vi "readInAoXML.vi"(8 "error in (no error)":errorcluster, 10 "NativeXML in":refnum<class "NativeXML.lvclass">, 11 "deviceDataBase in":refnum<class "deviceDataBase.lvclass">) -> (0 "error out":errorcluster, 1 "device.lvclass out":refnum<class "device.lvclass">, 3 "deviceDataBase out":refnum<class "deviceDataBase.lvclass">)   [LabVIEW 2011, in "Tools.lvlib" / "DatabaseHelpers.lvlib" / "deviceDataBase.lvclass"]
uses:
  deviceDataBase.lvclass
  NativeXML/NativeXML.lvclass
  Database Objects/device/device.lvclass
  Database Objects/device/AnalogDevice/AnalogDevice.lvclass
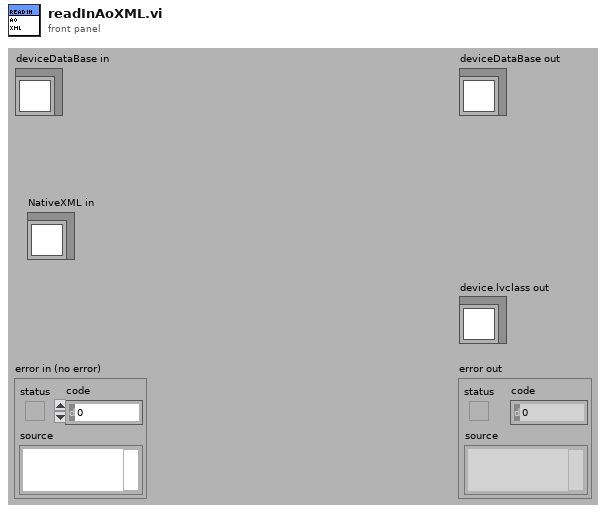
[diagram p1: front panel]
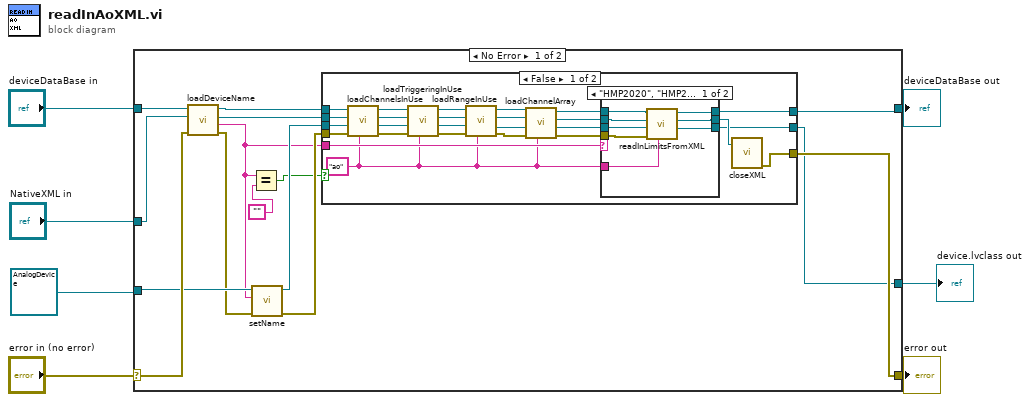
[diagram p0: block diagram]
diagram:
  n1 = case shown="No Error" "error in (no error)" {
    selector: "error in (no error)" -> [w21 w64]
    tunnel: [w13 w64] -> w6
    tunnel: [w12 w63] -> w4
    tunnel: "deviceDataBase in" -> [w22 w63]
    tunnel: "NativeXML in" -> [w20 _]
    tunnel: refnum<class "AnalogDevice.lvclass"> refnum ("Tools.lvlib:DatabaseHelpers.lvlib:AnalogDevice.lvclass") -> [w19 _]
    tunnel: [w9 _] -> w1
    frame No Error {
      n2 = call "loadDeviceName.vi"("error in (no error)"=w21, "NativeXML in"=w20, "deviceDataBase in"=w22) -> ("error out"=w18:errorcluster, "deviceName"=w8:string, "NativeXML out"=w15:refnum<class "NativeXML.lvclass">, "deviceDataBase out"=w17:refnum<class "deviceDataBase.lvclass">)  [unwired: 5 in]
      n3 = Equal?(x=w8, y="") -> (x = y?=w11:bool)
      n4 = call "setName.vi"("error in (no error)"=w18, "name"=w8, "device.lvclass in"=w19) -> ("error out"=w16:errorcluster, "device.lvclass out"=w14:refnum<class "AnalogDevice.lvclass">)  [unwired: 7 in]
      n5 = case shown="False" w11 {
        tunnel: w17 -> [w48 w62]
        tunnel: w16 -> [w47 w60]
        tunnel: w15 -> [w46 _]
        tunnel: w14 -> [w45 w61]
        tunnel: [w32 w60] -> w13
        tunnel: [w26 w61] -> w9
        tunnel: [w31 w62] -> w12
        tunnel: w8 -> [w25 _]
        frame False {
          w23 = "ao"
          n6 = call "loadChannelsInUse.vi"("type"=w23, "error in (no error)"=w47, "device.lvclass"=w45, "NativeXML in"=w46, "deviceDataBase in"=w48) -> ("error out"=w44:errorcluster, "device.lvclass out"=w41:refnum<class "device.lvclass">, "NativeXML out"=w42:refnum<class "NativeXML.lvclass">, "deviceDataBase out"=w43:refnum<class "deviceDataBase.lvclass">)  [unwired: 3 in]
          n7 = call "loadTriggeringInUse.vi"("type"=w23, "error in (no error)"=w44, "device.lvclass"=w41, "NativeXML in"=w42, "deviceDataBase in"=w43) -> ("error out"=w37:errorcluster, "device.lvclass out"=w38:refnum<class "device.lvclass">, "NativeXML out"=w39:refnum<class "NativeXML.lvclass">, "deviceDataBase out"=w40:refnum<class "deviceDataBase.lvclass">)  [unwired: 3 in]
          n8 = call "loadRangeInUse.vi"("type"=w23, "error in (no error)"=w37, "device.lvclass"=w38, "NativeXML in"=w39, "deviceDataBase in"=w40) -> ("error out"=w35:errorcluster, "device.lvclass out"=w33:refnum<class "device.lvclass">, "NativeXML out"=w34:refnum<class "NativeXML.lvclass">, "deviceDataBase out"=w36:refnum<class "deviceDataBase.lvclass">)  [unwired: 3 in]
          n9 = call "loadChannelArray.vi"("type"=w23, "error in (no error)"=w35, "device.lvclass"=w33, "NativeXML in"=w34, "deviceDataBase in"=w36) -> ("error out"=w24:errorcluster, "device.lvclass out"=w27:refnum<class "device.lvclass">, "NativeXML out"=w28:refnum<class "NativeXML.lvclass">, "deviceDataBase out"=w30:refnum<class "deviceDataBase.lvclass">)  [unwired: 3 in]
          n10 = case shown="\"HMP2020\", \"HMP2030\", \"HMP4030\"" w25 {
            tunnel: [w55 w59] -> w31
            tunnel: w30 -> [w56 w59]
            tunnel: [w54 w58] -> w29
            tunnel: w28 -> [w52 w58]
            tunnel: [w53 w57] -> w26
            tunnel: w27 -> [w51 w57]
            tunnel: w24 -> [w50 _]
            tunnel: w23 -> [w49 _]
            frame "HMP2020", "HMP2030", "HMP4030" {
              n11 = call "readInLimitsFromXML.vi"("type"=w49, "error in (no error)"=w50, "device.lvclass"=w51, "xml in"=w52, "deviceDataBase in"=w56) -> ("device.lvclass out"=w53:refnum<class "device.lvclass">, "xml out"=w54:refnum<class "NativeXML.lvclass">, "deviceDataBase out"=w55:refnum<class "deviceDataBase.lvclass">)  [unwired: 3 in, 1 out]
            }
            frame Default {
            }
          }
          n12 = call "closeXML.vi"("NativeXML in"=w29) -> ("error out"=w32:errorcluster)  [unwired: 10 in]
        }
        frame True {
        }
      }
    }
    frame Error {
    }
  }
  "error out" <- w6
  "deviceDataBase out" <- w4
  "device.lvclass out" <- w1
